vi "Cast.vi"(4 "Number of Shifts":i32, 6 "Lookup Table":sgl[](array[numeric]), 7 "Method":T1 items=["Use Bit Depth", "Shift", "Use Lookup Table"], 8 "error in":errorcluster, 9 "Image Type":T2, 10 "Image Dst Reference In":T3, 11 "Image Src Reference In":T3) -> (0 "error out":errorcluster, 3 "Image Dst Reference Out":T3)   [LabVIEW 2020, in "OpenLvVision_Image.lvlib" / "Management.lvlib"]
doc: "Converts the image's pixel data type."
uses:
  Management.lvlib
  TypeDef/Image.ctl
  TypeDef/ImageType.ctl
  TypeDef/CastMethode.ctl
  DataAccess/DataAccess.lvlib
  DLLs/OLV_VisionCore_AVX2_X86.dll
  DLLs/OLV_VisionCore_AVX2_X64.dll
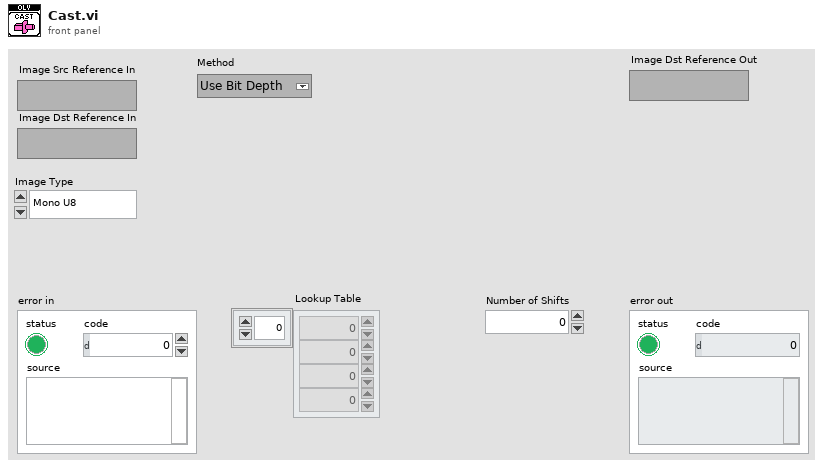
[diagram p1: front panel]
types:
  T1 = typedef "OpenLvVision_Image.lvlib/Management.lvlib/CastMethode.ctl" = u32
  T2 = typedef "OpenLvVision_Image.lvlib/Management.lvlib/ImageType.ctl" = enum16{"Mono U8", "Mono U16", "Mono I16", "Mono SGL", "Color U32", "Color U64", "Complex CSG"}
  T3 = typedef "OpenLvVision_Image.lvlib/Management.lvlib/Image.ctl" = refnum<image>
  T4 = typedef "OpenLvVision_Image.lvlib/DataAccess.lvlib/ImagePointer.ctl" = cluster{"ImagePointer":u64, "BorderSize":i32, "LineWidth":i32, "Width":i32, "Height":i32, "ImageFormat":T2}
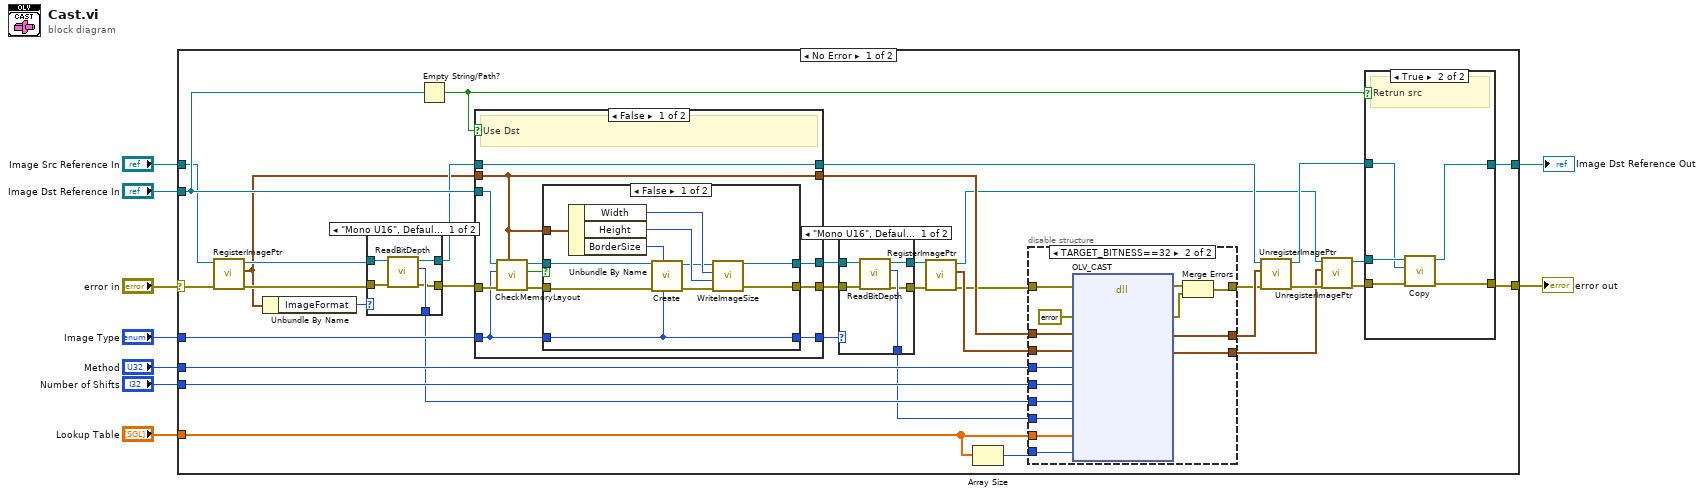
[diagram p0: block diagram]
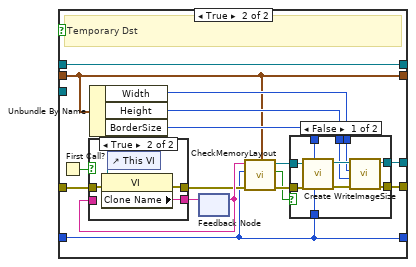
[diagram p4: hidden frame]
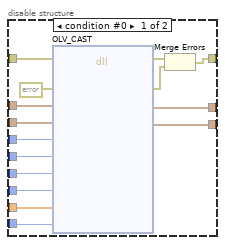
[diagram p8: hidden frame]
diagram:
  n1 = case shown="No Error" "error in" {
    selector: "error in" -> [w18 w156]
    tunnel: [w26 w156] -> w8
    tunnel: "Image Dst Reference In" -> [w34 _]
    tunnel: "Image Src Reference In" -> [w19 w157]
    tunnel: "Image Type" -> [w33 _]
    tunnel: "Lookup Table" -> [w44 _]
    tunnel: "Number of Shifts" -> [w43 _]
    tunnel: "Method" -> [w42 _]
    tunnel: [w36 w157] -> w1
    frame No Error {
      n2 = call "RegisterImagePtr.vi"("error in"=w18, "Image Reference In"=w19) -> ("error out"=w17:errorcluster, "ImagePointer"=w11:T4, "Image Reference Out"=w13:T3)  [unwired: 7 in]
      n3 = Unbundle By Name(w11) -> ("ImageFormat"=w10:T2)
      n4 = case shown="\"Mono U16\", Default" w10 {
        tunnel: w17 -> [w50 w51]
        tunnel: w13 -> [w49 w52]
        tunnel: [w48 w52] -> w12
        tunnel: [w47 _] -> w15
        tunnel: [w46 w51] -> w16
        frame "Mono U16", Default {
          n5 = call "ReadBitDepth.vi"("error in"=w50, "Image Reference In"=w49) -> ("error out"=w46:errorcluster, "BitDepth"=w47:u32, "Image Reference Out"=w48:T3)  [unwired: 7 in]
        }
        frame "Mono U8", "Color U32" {
        }
      }
      n6 = Empty String/Path?(string/path=w34) -> (empty?=w29:bool)
      n7 = case shown="False" w29 {
        tunnel: w16 -> [w62 w87]
        tunnel: [w57 w93] -> w24
        tunnel: w34 -> [w61 _]
        tunnel: w12 -> [w63 w91]
        tunnel: w33 -> [w54 w78]
        tunnel: [w56 w92] -> w23
        tunnel: [w63 w91] -> w32
        tunnel: w11 -> [w55 w79]
        tunnel: [w55 w79] -> w31
        tunnel: [w53 w78] -> w20
        frame False {
          # "Use Dst"
          n8 = call "CheckMemoryLayout.vi"("SrcPointer"=w55, "error in"=w62, "Format"=w54, "DstImage Reference"=w61) -> ("error out"=w60:errorcluster, "Same"=w59:bool, "DstImage Reference"=w58:T3)  [unwired: 5 in]
          n9 = case shown="False" w59 {
            tunnel: w60 -> [w73 w76]
            tunnel: w58 -> [w74 w77]
            tunnel: [w71 w76] -> w57
            tunnel: [w70 w77] -> w56
            tunnel: w54 -> [w64 w75]
            tunnel: w55 -> [w69 _]
            tunnel: [w64 w75] -> w53
            frame False {
              n10 = Unbundle By Name(w69) -> ("Width"=w66:i32, "Height"=w67:i32, "BorderSize"=w68:i32)
              n11 = call "Create.vi"("Image Type"=w64, "Border"=w68, "error in"=w73, "Image Name"=w74) -> ("error out"=w72:errorcluster, "Image Reference Out"=w65:T3)  [unwired: 6 in]
              n12 = call "WriteImageSize.vi"("error in"=w72, "Height"=w67, "Width"=w66, "Image Reference In"=w65) -> ("error out"=w71:errorcluster, "Image Reference Out"=w70:T3)  [unwired: 6 in]
            }
            frame True {
            }
          }
        }
        frame True {
          # "Temporary Dst"
          n13 = First Call?() -> (First Call?: T/F=w86:bool)
          n14 = Unbundle By Name(w79) -> ("Width"=w90:i32, "Height"=w89:i32, "BorderSize"=w88:i32)
          n15 = feedback #1() -> (w84:string)  [unwired: 1 in]
          n16 = case shown="True" w86 {
            tunnel: w87 -> [w107 w111]
            tunnel: [w107 w110] -> w83
            tunnel: [w106 w109] -> w85
            tunnel: w84 -> [w106 _]
            frame False {
            }
            frame True {
              n17 = control-ref of="This VI"() -> (w108:refnum<vi>)
              n18 = property class="VI"(reference=w108, error in=w111) -> (error out=w110:errorcluster, "Clone Name"=w109:string)  [unwired: 1 out]
            }
          }
          n19 = feedback-in #1(w85) -> ()
          n20 = call "CheckMemoryLayout.vi"("SrcPointer"=w79, "error in"=w83, "Format"=w78, "DstImage Reference"=w84) -> ("error out"=w82:errorcluster, "Same"=w80:bool, "DstImage Reference"=w81:T3)  [unwired: 5 in]
          n21 = case shown="False" w80 {
            tunnel: [w102 w104] -> w93
            tunnel: w78 -> [w101 _]
            tunnel: [w99 w105] -> w92
            tunnel: w90 -> [w98 _]
            tunnel: w89 -> [w97 _]
            tunnel: w88 -> [w96 _]
            tunnel: w82 -> [w95 w104]
            tunnel: w81 -> [w94 w105]
            frame False {
              n22 = call "Create.vi"("Image Type"=w101, "Border"=w96, "error in"=w95, "Image Name"=w94) -> ("error out"=w103:errorcluster, "Image Reference Out"=w100:T3)  [unwired: 6 in]
              n23 = call "WriteImageSize.vi"("error in"=w103, "Height"=w97, "Width"=w98, "Image Reference In"=w100) -> ("error out"=w102:errorcluster, "Image Reference Out"=w99:T3)  [unwired: 6 in]
            }
            frame True {
            }
          }
        }
      }
      n24 = case shown="\"Mono U16\", Default" w20 {
        tunnel: w24 -> [w116 w117]
        tunnel: w23 -> [w115 w118]
        tunnel: [w114 w118] -> w22
        tunnel: [w113 _] -> w14
        tunnel: [w112 w117] -> w21
        frame "Mono U16", Default {
          n25 = call "ReadBitDepth.vi"("error in"=w116, "Image Reference In"=w115) -> ("error out"=w112:errorcluster, "BitDepth"=w113:u32, "Image Reference Out"=w114:T3)  [unwired: 7 in]
        }
        frame "Mono U8", "Color U32" {
        }
      }
      n26 = call "RegisterImagePtr.vi"("error in"=w21, "Image Reference In"=w22) -> ("error out"=w25:errorcluster, "ImagePointer"=w35:T4, "Image Reference Out"=w30:T3)  [unwired: 7 in]
      n27 = Array Size(array=w44) -> (size(s)=w45:i32)
      n28 = disable-structure shown="TARGET_BITNESS==32" {
        disable-tunnel: w45 -> [w133 w148]
        disable-tunnel: w44 -> [w132 w147]
        disable-tunnel: w43 -> [w131 w146]
        disable-tunnel: w42 -> [w130 w145]
        disable-tunnel: [w121 w137] -> w28
        disable-tunnel: [w129 w144] -> w40
        disable-tunnel: [w128 w143] -> w39
        disable-tunnel: w25 -> [w127 w142]
        disable-tunnel: w35 -> [w126 w141]
        disable-tunnel: w31 -> [w125 w140]
        disable-tunnel: w15 -> [w120 w135]
        disable-tunnel: w14 -> [w119 w134]
        frame condition #0 {
          n29 = dll-call lib="C:/Users/lukas/Downloads/OpenLvVision_Image/SourceCode/DLLs/OLV_VisionCore_AVX2_X64.dll" fn="OLV_CAST"(error in=w127, "Error"=errorcluster {"status"=FALSE, "code"=0, "source"=""} ("error out"), "SrcImageInfo"=w125, "DstImageInfo"=w126, "Methode"=w130, "NumberOfShifts"=w131, "bitdepthSrc"=w120, "bitdepthDst"=w119, "LookupTable"=w132, "LookupTableSize"=w133) -> (error out=w123:errorcluster, "Error"=w122:errorcluster, "SrcImageInfo"=w129:T4, "DstImageInfo"=w128:T4)  [unwired: 9 in, 1 out]
          n30 = Merge Errors(w123, w122) -> (w121:errorcluster)
        }
        frame condition #1 (active) {
          n31 = dll-call lib="C:/Users/lukas/Downloads/OpenLvVision_Image/SourceCode/DLLs/OLV_VisionCore_AVX2_X86.dll" fn="OLV_CAST"(error in=w142, "Error"=errorcluster {"status"=FALSE, "code"=0, "source"=""} ("error out"), "SrcImageInfo"=w140, "DstImageInfo"=w141, "Methode"=w145, "NumberOfShifts"=w146, "bitdepthSrc"=w135, "bitdepthDst"=w134, "LookupTable"=w147, "LookupTableSize"=w148) -> (error out=w138:errorcluster, "Error"=w136:errorcluster, "SrcImageInfo"=w144:T4, "DstImageInfo"=w143:T4)  [unwired: 9 in, 1 out]
          n32 = Merge Errors(w138, w136) -> (w137:errorcluster)
        }
      }
      n33 = call "UnregisterImagePtr.vi"("error in"=w28, "ImagePointer"=w40, "Image Reference In"=w32) -> ("error out"=w41:errorcluster, "Image Reference Out"=w37:T3)  [unwired: 7 in]
      n34 = call "UnregisterImagePtr.vi"("error in"=w41, "ImagePointer"=w39, "Image Reference In"=w30) -> ("error out"=w27:errorcluster, "Image Reference Out"=w38:T3)  [unwired: 7 in]
      n35 = case shown="True" w29 {
        tunnel: w27 -> [w149 w155]
        tunnel: w38 -> [w150 w153]
        tunnel: w37 -> [_ w152]
        tunnel: [w150 w154] -> w36
        tunnel: [w149 w151] -> w26
        frame False {
          # "Return Dst"
        }
        frame True {
          # "Retrun src"
          n36 = call "Copy.vi"("error in"=w155, "Image Dst Reference In"=w152, "Image Src Reference In"=w153) -> ("error out"=w151:errorcluster, "Image Dst Reference Out"=w154:T3)  [unwired: 7 in]
        }
      }
    }
    frame Error {
    }
  }
  "error out" <- w8
  "Image Dst Reference Out" <- w1
